vi "AuMT8852B EUT HCI RS232 Baud Rate.vi"(5 "Baud rate (1200)":T1(ring), 7 "Set/Get (Set)":enum16{"Set", "Get"}(ring), 8 "error in (no error)":errorcluster, 11 "VISA session":refnum<visa-resource-name>) -> (0 "error out":errorcluster, 2 "error code":i32, 3 "VISA session out":refnum<visa-resource-name>, 4 "Baud rate out":T1(ring))   [LabVIEW 2017]
doc: "Anritsu MT8852B Bluetooth Tester\n\nSets the baud rate of the HCI serial connection to the EUT.\n\nINPUTS\nSet/Get - whether the value is being sent to or retrieved from the instrument.\nBaud rate - rate to send to the instrument.\n\nOUTPUTS\nBaud rate out - the present baud rate being used by the instrument."
uses:
  <instrlib>/aumt8852B/General/Utilities/MT8850 Attribute ID.ctl
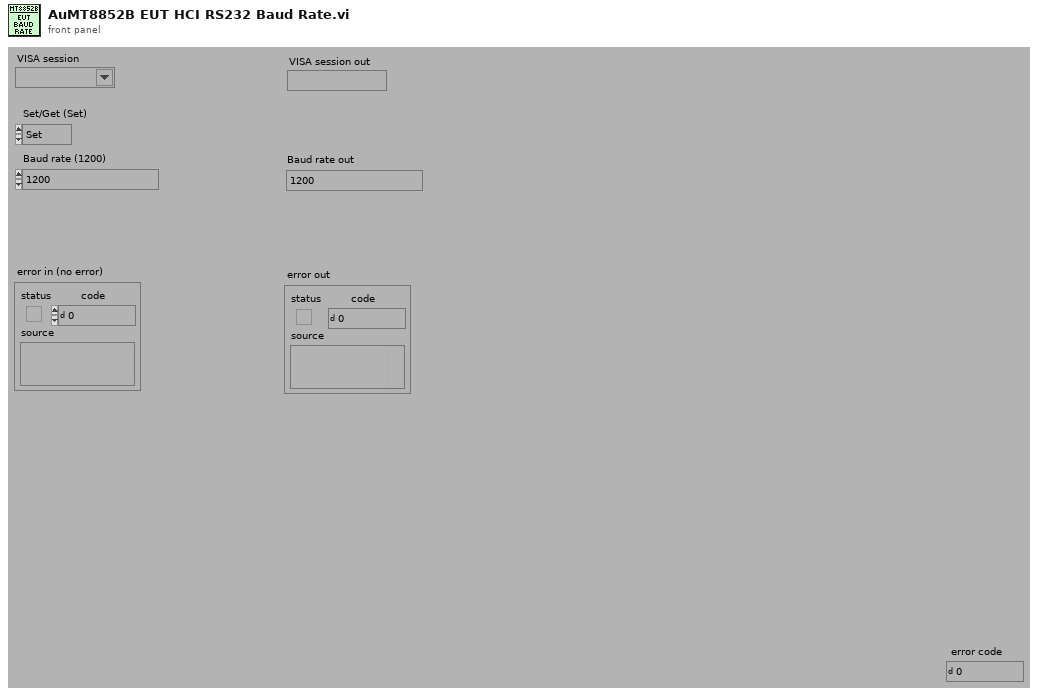
[diagram p1: front panel]
types:
  T1 = enum16{"1200", "2400", "4800", "9600", "19200", "38400", "57600", "115200", "230400", "460800", "921600"}
  T2 = typedef "MT8850 Attribute ID.ctl" = enum16{"Operation mode", "Selected script", "EUT address source", "EUT Address", "EUT HCI RS232 Baud Rate", "Tester GPIB Address", "Tester RS232 Baud Rate", "Tester Bluetooth Address", "Tester Contrast", "Tester Key Click On", "Tester Modulation Index", "Tester Poll-Null Mode", "Tester Power Range", "Tester RS232 Mode", "Beep on Illegal Entry", "Display User Text", "User Text", "Calibration TX Modulation DAC", "Calibration RX Channel", "Calibration TX Channel", "Calibration TX Power", "Calibration Use TX Table", "Inquiry Request User-friendly Name", "Inquiry Number of Responses", "Inquiry Timeout", "Script Frequency Display", "Script Loop Count", "Script Loop Continuously", "Script Loop Stop on Fail", "Link timeout", "Page timeout", "Filter bandwidth", "SCO air code", "SCO bit position", "SCO input code", "SCO input data", "SCO input sample size", "SCO loopback mode", "SCO packet type", "SCO tone generator", "Tester page scan repetition mode", "Tester follow test mode", "Tester authentication state", "Tester authentication pin code", "Tester authentication pin length"}
  T3 = typedef "Attribute Status.ctl" = enum16{"No I/O needed", "I/O needed"}
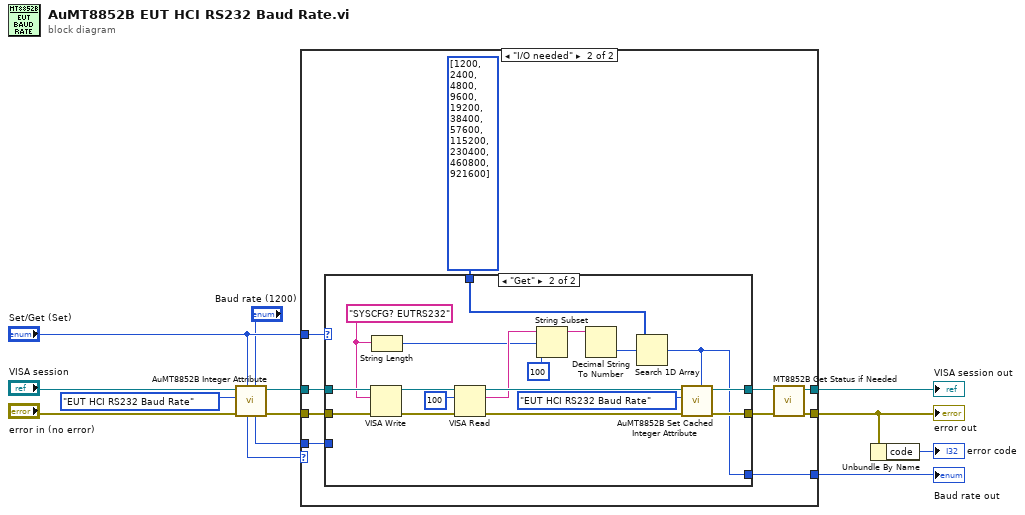
[diagram p0: block diagram]
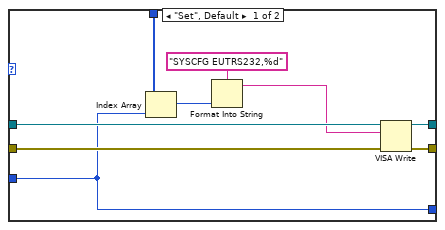
[diagram p3: hidden frame]
diagram:
  n1 = call <instrlib>:"AuMT8852B Integer Attribute.vi"("Value (0)"="Baud rate (1200)", "Set/Get (Set)"="Set/Get (Set)", "error in (no error)"="error in (no error)", "Attribute ID"=MT8850_Attribute_ID."EUT HCI RS232 Baud Rate", "VISA session"="VISA session") -> ("error out"=w6:errorcluster, "VISA session out"=w7:refnum<visa-resource-name>, "Value out"=w9:i32, "Status"=w4:T3)  [unwired: 3 in]
  n2 = case shown="\"I/O needed\"" w4 {
    tunnel: "Set/Get (Set)" -> [_ w26]
    tunnel: w9 -> [w16 w25]
    tunnel: [w14 w18] -> w1
    tunnel: [w15 w19] -> w8
    tunnel: w7 -> [w15 w24]
    tunnel: w6 -> [w14 w23]
    tunnel: [w16 w22] -> w3
    frame "No I/O needed", Default {
    }
    frame "I/O needed" {
      n3 = case shown="\"Get\"" w26 {
        tunnel: [w31 w45] -> w20
        tunnel: w25 -> [w33 _]
        tunnel: [w32 w46] -> w21
        tunnel: w24 -> [w35 w53]
        tunnel: w23 -> [w34 w52]
        tunnel: [w33 w44] -> w22
        tunnel: i32[] [1200, 2400, 4800, 9600, 19200, 38400, 57600, 115200, 230400, 460800, 921600] ("Array Constant") -> [w29 w39]
        frame "Set", Default {
          n4 = Index Array(array=w29, index=w33) -> (element=w28:i32)
          n5 = Format Into String(format string="SYSCFG EUTRS232,%d" ("Substring"), w28) -> (resulting string=w27:string)  [unwired: 2 in, 1 out]
          n6 = VISA Write(VISA resource name=w35, write buffer=w27, error in (no error)=w34) -> (VISA resource name out=w32:refnum<visa-resource-name>, error out=w31:errorcluster)  [unwired: 1 out]
        }
        frame "Get" {
          w38 = "SYSCFG? EUTRS232" ("write buffer (\"\")")
          n7 = VISA Write(VISA resource name=w53, write buffer=w38, error in (no error)=w52) -> (VISA resource name out=w51:refnum<visa-resource-name>, error out=w49:errorcluster)  [unwired: 1 out]
          n8 = String Length(string=w38) -> (length=w37:i32)
          n9 = VISA Read(VISA resource name=w51, byte count=u32 100 ("byte count (0)"), error in (no error)=w49) -> (VISA resource name out=w48:refnum<visa-resource-name>, read buffer=w42:string, error out=w47:errorcluster)  [unwired: 1 out]
          n10 = String Subset(string=w42, offset (0)=w37, length (rest)=100 ("length (rest)")) -> (substring=w41:string)
          n11 = Decimal String To Number(string=w41) -> (number=w40:i32)  [unwired: 2 in, 1 out]
          n12 = Search 1D Array(1D array=w39, element=w40) -> (index of element=w44:i32)  [unwired: 1 in]
          n13 = call <instrlib>:"AuMT8852B Set Cached Integer Attribute.vi"("Value (0)"=w44, "error in (no error)"=w47, "Attribute ID"=MT8850_Attribute_ID."EUT HCI RS232 Baud Rate", "VISA session"=w48) -> ("error out"=w45:errorcluster, "VISA session out"=w46:refnum<visa-resource-name>)  [unwired: 6 in]
        }
      }
      n14 = call <instrlib>:"MT8852B Get Status if Needed.vi"("error in (no error)"=w20, "VISA session"=w21) -> ("error out"=w18:errorcluster, "VISA session out"=w19:refnum<visa-resource-name>)  [unwired: 8 in]
    }
  }
  "error out" <- w1
  "VISA session out" <- w8
  "Baud rate out" <- w3
  n15 = Unbundle By Name(w1) -> ("code"=→"error code":i32)
